vi "AH_V_to_C.vi"(11 "Vin[1-5V]":dbl) -> (3 "Tout[C]":dbl)   [LabVIEW 2019]
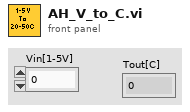
[diagram p1: front panel]
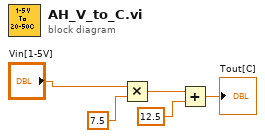
[diagram p0: block diagram]
diagram:
  n1 = Multiply(x="Vin[1-5V]", y=7.5) -> (x*y=w4:dbl)
  n2 = Add(x=w4, y=12.5) -> (x+y=→"Tout[C]":dbl)
